vi "Show Windows.vi"(7 "nCmdShow":string(combo), 8 "error in (no error)":errorcluster, 11 "hWnd":u32) -> (0 "error out":errorcluster, 3 "hWnd out":u32)   [LabVIEW 2019, in "Test Bench Tools.lvlib"]
uses:
  Test Bench Tools.lvlib
  user32.dll
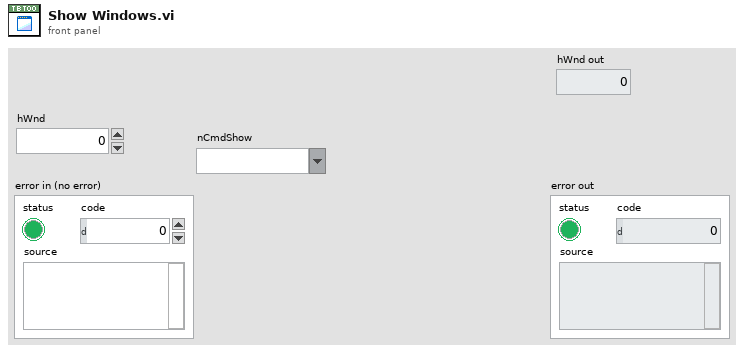
[diagram p1: front panel]
types:
  T1 = enum16{"SW_HIDE", "SW_SHOWNORMAL", "SW_SHOWMINIMIZED", "SW_MAXIMIZE", "SW_SHOWNOACTIVATE", "SW_SHOW", "SW_MINIMIZE", "SW_SHOWMINNOACTIVE", "SW_SHOWNA", "SW_RESTORE", "SW_SHOWDEFAULT"}
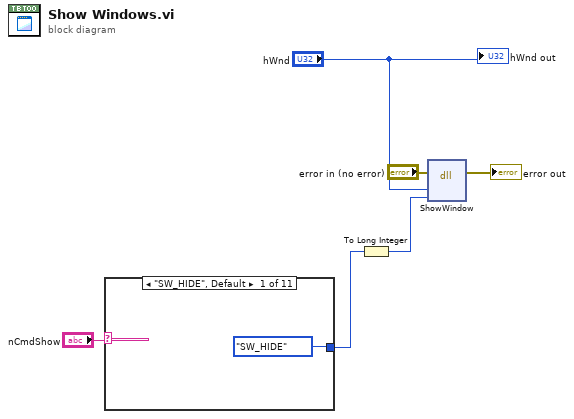
[diagram p0: block diagram]
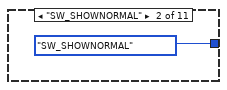
[diagram p2: hidden frame]
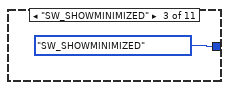
[diagram p3: hidden frame]
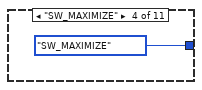
[diagram p4: hidden frame]
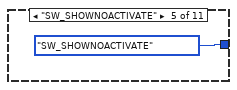
[diagram p5: hidden frame]
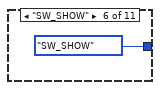
[diagram p6: hidden frame]
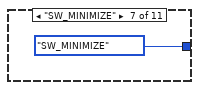
[diagram p7: hidden frame]
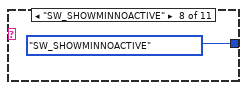
[diagram p8: hidden frame]
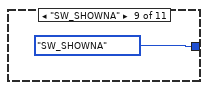
[diagram p9: hidden frame]
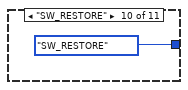
[diagram p10: hidden frame]
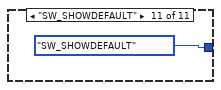
[diagram p11: hidden frame]
diagram:
  n1 = case shown="\"SW_HIDE\", Default" "nCmdShow" {
    tunnel: [T1."SW_HIDE" ("nCmdShow") T1."SW_SHOWNORMAL" ("nCmdShow") T1."SW_SHOWMINIMIZED" ("nCmdShow") T1."SW_MAXIMIZE" ("nCmdShow") T1."SW_SHOWNOACTIVATE" ("nCmdShow") T1."SW_SHOW" ("nCmdShow") T1."SW_MINIMIZE" ("nCmdShow") T1."SW_SHOWMINNOACTIVE" ("nCmdShow") T1."SW_SHOWNA" ("nCmdShow") T1."SW_RESTORE" ("nCmdShow") T1."SW_SHOWDEFAULT" ("nCmdShow")] -> w1
    frame "SW_HIDE", Default {
    }
    frame "SW_SHOWNORMAL" {
    }
    frame "SW_SHOWMINIMIZED" {
    }
    frame "SW_MAXIMIZE" {
    }
    frame "SW_SHOWNOACTIVATE" {
    }
    frame "SW_SHOW" {
    }
    frame "SW_MINIMIZE" {
    }
    frame "SW_SHOWMINNOACTIVE" {
    }
    frame "SW_SHOWNA" {
    }
    frame "SW_RESTORE" {
    }
    frame "SW_SHOWDEFAULT" {
    }
  }
  n2 = To Long Integer(number=w1) -> (32bit integer=w3:i32)
  n3 = dll-call lib="user32.dll" fn="ShowWindow"(error in="error in (no error)", "hWnd"="hWnd", "nCmdShow"=w3) -> (error out=→"error out":errorcluster)  [unwired: 5 in, 1 out]
  "hWnd out" <- "hWnd"
